vi "Evaluate Method Status.vi"(11 "Results":T2[](array[typedef])) -> (3 "Status":T1=enum."Passed")   [LabVIEW 2020, in "LUnit Test Case.lvclass"]
uses:
  LUnit Test Case.lvclass
  Core/Result/Result.ctl
  Core/Result/Status.ctl
  Core/Result/Type.ctl
  Core/Result/Result.lvlib
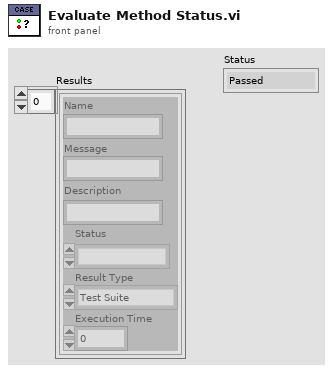
[diagram p1: front panel]
types:
  T1 = typedef "Result.lvlib/Status.ctl" = enum16{"", "Passed", "Failed", "Error", "Skipped", "Setup Error", "Broken", "Teardown Error"}
  T2 = typedef "Result.lvlib/Result.ctl" = cluster{"Name":string, "Message":string, "Description":string, "Status":T1, "Result Type":T3, "Execution Time":dbl}
  T3 = typedef "Result.lvlib/Type.ctl" = enum16{"Test Case", "Test Suite", "Test Run", "Pass", "Fail", "Skip", "Pass if", "Fail if", "Pass if Error", "Fail if Error", "Pass if Equal", "Fail if Equal"}
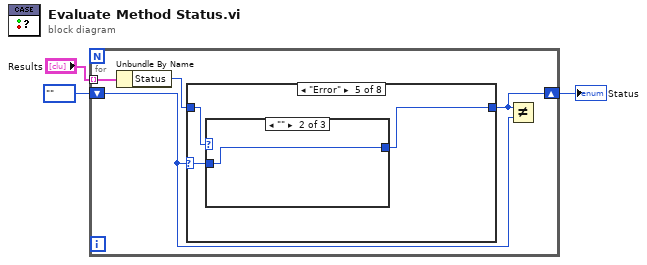
[diagram p0: block diagram]
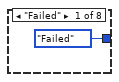
[diagram p3: hidden frame]
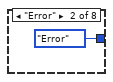
[diagram p4: hidden frame]
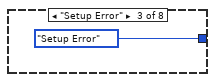
[diagram p5: hidden frame]
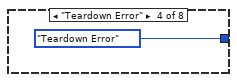
[diagram p6: hidden frame]
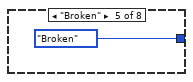
[diagram p7: hidden frame]
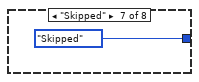
[diagram p8: hidden frame]
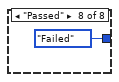
[diagram p9: hidden frame]
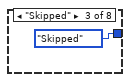
[diagram p11: hidden frame]
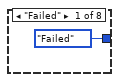
[diagram p13: hidden frame]
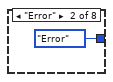
[diagram p14: hidden frame]
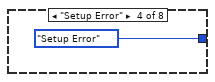
[diagram p15: hidden frame]
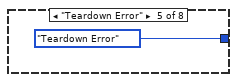
[diagram p16: hidden frame]
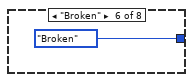
[diagram p17: hidden frame]
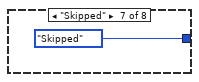
[diagram p18: hidden frame]
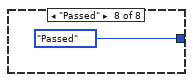
[diagram p19: hidden frame]
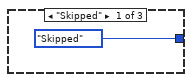
[diagram p20: hidden frame]
diagram:
  n1 = for {
    tunnel: "Results" -> [w7] mode=indexing
    shift-right: [w5] -> w1
    shift-left: Status."" ("Current") -> [w6]
    n2 = Unbundle By Name(w7) -> ("Status"=w4:T1)
    n3 = case shown="\"Error\"" w6 {
      selector: w6 -> [w8 _ _ w21 w32 _ _ _]
      tunnel: w4 -> [w10 w19 _ w23 w33 w38 w42 w46]
      tunnel: [w9 w19 Status."Skipped" ("Merged Status") w22 w34 w39 w43 w47] -> w5
      frame "Failed" {
        n4 = case shown="\"\"" w10 {
          tunnel: [Status."Failed" ("Merged Status") Status."Error" ("Merged Status") Status."Setup Error" ("Merged Status") Status."Teardown Error" ("Merged Status") Status."Broken" ("Merged Status") w16 Status."Skipped" ("Merged Status") Status."Failed" ("Merged Status")] -> w9
          tunnel: w8 -> [_ _ _ _ _ w16 _ _]
          frame "Failed" {
          }
          frame "Error" {
          }
          frame "Setup Error" {
          }
          frame "Teardown Error" {
          }
          frame "Broken" {
          }
          frame "" {
          }
          frame "Skipped" {
          }
          frame "Passed" {
          }
        }
      }
      frame "" {
      }
      frame "Skipped" {
      }
      frame "Passed" {
        n5 = case shown="\"\"" w23 {
          tunnel: [Status."Failed" ("Merged Status") Status."Error" ("Merged Status") w26 Status."Setup Error" ("Merged Status") Status."Teardown Error" ("Merged Status") Status."Broken" ("Merged Status") Status."Skipped" ("Merged Status") Status."Passed" ("Merged Status")] -> w22
          tunnel: w21 -> [_ _ w26 _ _ _ _ _]
          frame "Failed" {
          }
          frame "Error" {
          }
          frame "" {
          }
          frame "Setup Error" {
          }
          frame "Teardown Error" {
          }
          frame "Broken" {
          }
          frame "Skipped" {
          }
          frame "Passed" {
          }
        }
      }
      frame "Error" {
        n6 = case shown="\"\"" w33 {
          tunnel: [Status."Skipped" ("Merged Status") w36 Status."Error" ("Merged Status")] -> w34
          tunnel: w32 -> [_ w36 _]
          frame "Skipped" {
          }
          frame "" {
          }
          frame Default {
          }
        }
      }
      frame "Setup Error" {
        n7 = case shown="Default" w38 {
          tunnel: [Status."Skipped" ("Merged Status") Status."Setup Error" ("Merged Status")] -> w39
          frame "Skipped" {
          }
          frame Default {
          }
        }
      }
      frame "Broken" {
        n8 = case shown="Default" w42 {
          tunnel: [Status."Broken" ("Merged Status") Status."Setup Error" ("Merged Status")] -> w43
          frame Default {
          }
          frame "Setup Error" {
          }
        }
      }
      frame "Teardown Error" {
        n9 = case shown="Default" w46 {
          tunnel: [Status."Skipped" ("Merged Status") Status."Teardown Error" ("Merged Status")] -> w47
          frame "Skipped" {
          }
          frame Default {
          }
        }
      }
    }
    n10 = Not Equal?(x=w5, y=w6) -> ()  [unwired: 1 out]
  }
  "Status" <- w1
